vi "Read Ramp visible.vi"(9 "ColorScale in":refnum<class "ColorScale.lvclass">) -> (3 "ColorScale out":refnum<class "ColorScale.lvclass">, 4 "Ramp visible":bool)   [LabVIEW 2014, in "ColorScale.lvclass"]
uses:
  ColorScale.lvclass
  ColorScale.lvclass/ColorScale.ctl
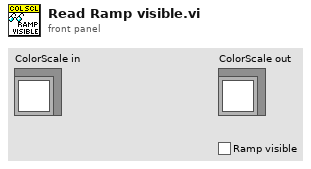
[diagram p1: front panel]
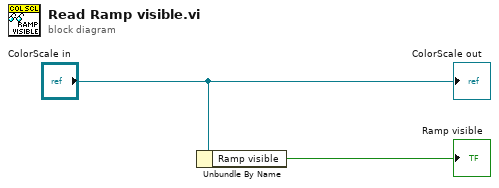
[diagram p0: block diagram]
diagram:
  n1 = Unbundle By Name("ColorScale in") -> ("Ramp visible"=→"Ramp visible":bool)
  "ColorScale out" <- "ColorScale in"
